vi "Teleop.vi"(10 "Match Info":T2={"Autonomous Elapsed Seconds"=0.0, "TeleOp Elapsed Seconds"=0.0, "Disabled Elapsed Seconds"=0.0, "Visited Autonomous"=FALSE, "Visited TeleOp"=FALSE, "Visited Disabled"=FALSE, "Autonomous Settings"={"Autonomous Style"=enum."Independent", "VI Refnum"=refnum}}, 11 "Call Context":T3) -> ()   [LabVIEW 2017]
doc: "This VI is called for each TeleOp packet received from the DS where the robot is not disabled. It is often used to read from the joysticks and update I/O or to update setpoints for timed control loops. It should complete and return within 20 milliseconds or it may miss DS packets."
uses:
  <vilib>/Rock Robotics/WPI/DriverStation/WPI_DriverStationDerivedRobotMode.ctl
  <vilib>/Rock Robotics/WPI/DriverStation/WPI_DriverStationMatch Info.ctl
  <vilib>/Rock Robotics/WPI/Solenoid/WPI_SolenoidValue.ctl
  <vilib>/Rock Robotics/WPI/Utilities/WPI_GetSetVariantRefNum.vi
  <vilib>/Rock Robotics/WPI/Solenoid/WPI_SolenoidSetEnum.vi
  <vilib>/Rock Robotics/WPI/RobotDrive/WPI_RobotDriveMecanumDrive_Cartesian.vi
  <vilib>/Rock Robotics/Network Tables/NT Write Numeric Array.vi
  <vilib>/Rock Robotics/Network Tables/NT Write Number.vi
  Robot Global Data.vi
panel:
  out "Stopped":bool
  out "Rate":dbl
  out "Direction":bool
  out "Distance":dbl
  out "Accelerations":T1
  out "Switch Pressed":bool
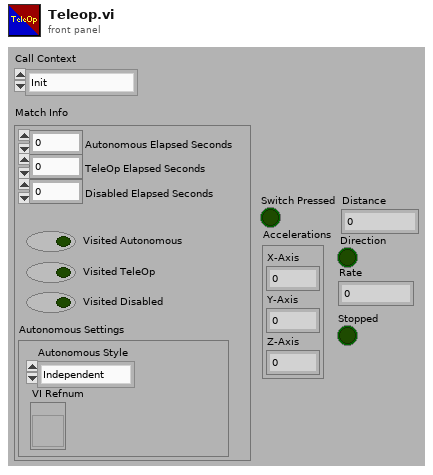
[diagram p1: front panel]
types:
  T1 = cluster{"X-Axis":dbl, "Y-Axis":dbl, "Z-Axis":dbl}
  T2 = typedef "WPI_DriverStationMatch Info.ctl" = cluster{"Autonomous Elapsed Seconds":dbl, "TeleOp Elapsed Seconds":dbl, "Disabled Elapsed Seconds":dbl, "Visited Autonomous":bool, "Visited TeleOp":bool, "Visited Disabled":bool, "Autonomous Settings":cluster{"Autonomous Style":enum16{"Iterative", "Independent"}, "VI Refnum":refnum<vi>}}
  T3 = typedef "WPI_DriverStationDerivedRobotMode.ctl" = enum16{"Init", "Execute", "Stop"}
  T4 = typedef "WPI_RobotDriveDevRef.ctl" = cluster{"DevStatus":errorcluster, "Motors[]":T5[], "Square Inputs":bool, "Max Output":dbl}
  T5 = typedef "WPI_MotorControlDeviceRef.ctl" = cluster{"DeviceStatus":errorcluster, "Type":T6, "PWM":cluster{"PWM Channel":T7, "DeadBand":T8}, "CAN":cluster{"Device Number":u8, "SetOutput VI Ref":variant, "GetOutput VI Ref":variant, "Enable VI Ref":variant, "Disable VI Ref":variant, "Data":variant}, "Invert":bool, "DIO PWM":cluster{"PWM \"Enable\" Channel":T7, "DIOChannel":T9, "PWM Rate":dbl}}
  T6 = typedef "WPI_MotorControlType.ctl" = enum16{"PWM", "CAN", "DIO PWM"}
  T7 = typedef "FPGA_DIOPWMChannel.ctl" = enum8{"PWM 0", "PWM 1", "PWM 2", "PWM 3", "PWM 4", "PWM 5", "PWM 6", "PWM 7", "PWM 8", "PWM 9", "PWM MXP 0", "PWM MXP 1", "PWM MXP 2", "PWM MXP 3", "PWM MXP 4", "PWM MXP 5", "PWM MXP 6", "PWM MXP 7", "PWM MXP 8", "PWM MXP 9", "Invalid"}
  T8 = typedef "WPI_PWMDeadband.ctl" = cluster{"Name":string, "maxPositivePwm":i32, "minPositivePwm":i32, "centerPwm":i32, "maxNegativePwm":i32, "minNegativePwm":i32, "angularRange":u16}
  T9 = typedef "FPGA_DIOChannel.ctl" = enum8{"DIO 0", "DIO 1", "DIO 2", "DIO 3", "DIO 4", "DIO 5", "DIO 6", "DIO 7", "DIO 8", "DIO 9", "DIO MXP 0", "DIO MXP 1", "DIO MXP 2", "DIO MXP 3", "DIO MXP 4", "DIO MXP 5", "DIO MXP 6", "DIO MXP 7", "DIO MXP 8", "DIO MXP 9", "DIO MXP 10", "DIO MXP 11", "DIO MXP 12", "DIO MXP 13", "DIO MXP 14", "DIO MXP 15", "SPI Port CS1", "SPI Port CS2", "SPI Port CS3", "SPI Port MISO", "SPI Port MOSI", "Invalid"}
  T10 = typedef "WPI_JoystickDevRef.ctl" = cluster{"Device":T11}
  T11 = typedef "WPI_JoystickDeviceEnum.ctl" = enum16{"USB 0", "USB 1", "USB 2", "USB 3", "USB 4", "USB 5"}
  T12 = typedef "WPI_SolenoidValue.ctl" = enum16{"Off", "On", "Forward", "Reverse"}
  T13 = typedef "WPI_SolenoidDevRef.ctl" = cluster{"DevStatus":errorcluster, "Pneumatics Control Module":u8, "Forward Solenoid Channel":T14, "Reverse Solenoid Channel":T14}
  T14 = typedef "WPI_SolenoidChannel.ctl" = enum8{"Solenoid 0", "Solenoid 1", "Solenoid 2", "Solenoid 3", "Solenoid 4", "Solenoid 5", "Solenoid 6", "Solenoid 7", "Invalid"}
  T15 = typedef "WPI_SwitchDevRef.ctl" = cluster{"DevStatus":errorcluster, "DIO Channel":T9, "CntIndex":T16, "Normally Closed":bool}
  T16 = typedef "FPGA_CounterCtrSystemIndex.ctl" = enum8{"Ctr 0", "Ctr 1", "Ctr 2", "Ctr 3", "Ctr 4", "Ctr 5", "Ctr 6", "Ctr 7", "Invalid"}
  T17 = typedef "WPI_AccelerometerDevRef.ctl" = cluster{"DevStatus":errorcluster, "Scaling":T18, "Analog Channels":T19, "I2C Bus":T21, "SPI Bus":T22, "Accel Range":T23, "ADXL Axes":T24, "Handle":i32, "Device Address":u8, "Accel Type":enum16{"Analog", "ADXL345 I2C", "ADXL345 SPI", "Internal", "ADXL362 SPI"}}
  T18 = typedef "WPI_AccelerometerScaling.ctl" = cluster{"Gain (VoltsPerG)":dbl, "Center Voltage":dbl}
  T19 = typedef "WPI_AccelerometerAnalogChannels.ctl" = cluster{"X-Axis":T20, "Y-Axis":T20, "Z-Axis":T20}
  T20 = typedef "FPGA_AIChannel.ctl" = enum8{"AI 0", "AI 1", "AI 2", "AI 3", "AI MXP 0", "AI MXP 1", "AI MXP 2", "AI MXP 3", "Invalid"}
  T21 = typedef "i2c_bus.ctl" = enum16{"I2C On-Board", "I2C MXP", "Invalid"}
  T22 = typedef "spi_bus.ctl" = enum16{"SPI On-Board, CS0", "SPI On-Board, CS1", "SPI On-Board, CS2", "SPI On-Board, CS3", "SPI MXP", "Invalid"}
  T23 = typedef "ADXL345 Range.ctl" = u8
  T24 = typedef "WPI_AccelerometerADXL345 Axes.ctl" = cluster{"X-Axis":bool, "Y-Axis":bool, "Z-Axis":bool}
  T25 = typedef "WPI_EncoderDevRef.ctl" = cluster{"DevStatus":errorcluster, "EncoderIndex":T26, "CounterIndex":T16, "DistancePerCount":dbl, "Decoding Type":T27}
  T26 = typedef "FPGA_EncoderIdx.ctl" = enum8{"Enc 0", "Enc 1", "Enc 2", "Enc 3", "Enc 4", "Enc 5", "Enc 6", "Enc 7", "Invalid"}
  T27 = typedef "WPI_EncoderType.ctl" = enum16{"1x", "2x", "4x"}
  T28 = typedef "WPI_GyroDevRef.ctl" = cluster{"DevStatus":errorcluster, "Analog Channel":T20, "Gain (VoltsPerDegree/Second)":dbl, "Gyro Type":enum16{"Analog", "XRS450"}, "Handle":i32, "SPI Bus":T22, "Device Found":bool, "Sample Rate":dbl, "Calibrate On Open":bool, "Offset":dbl}
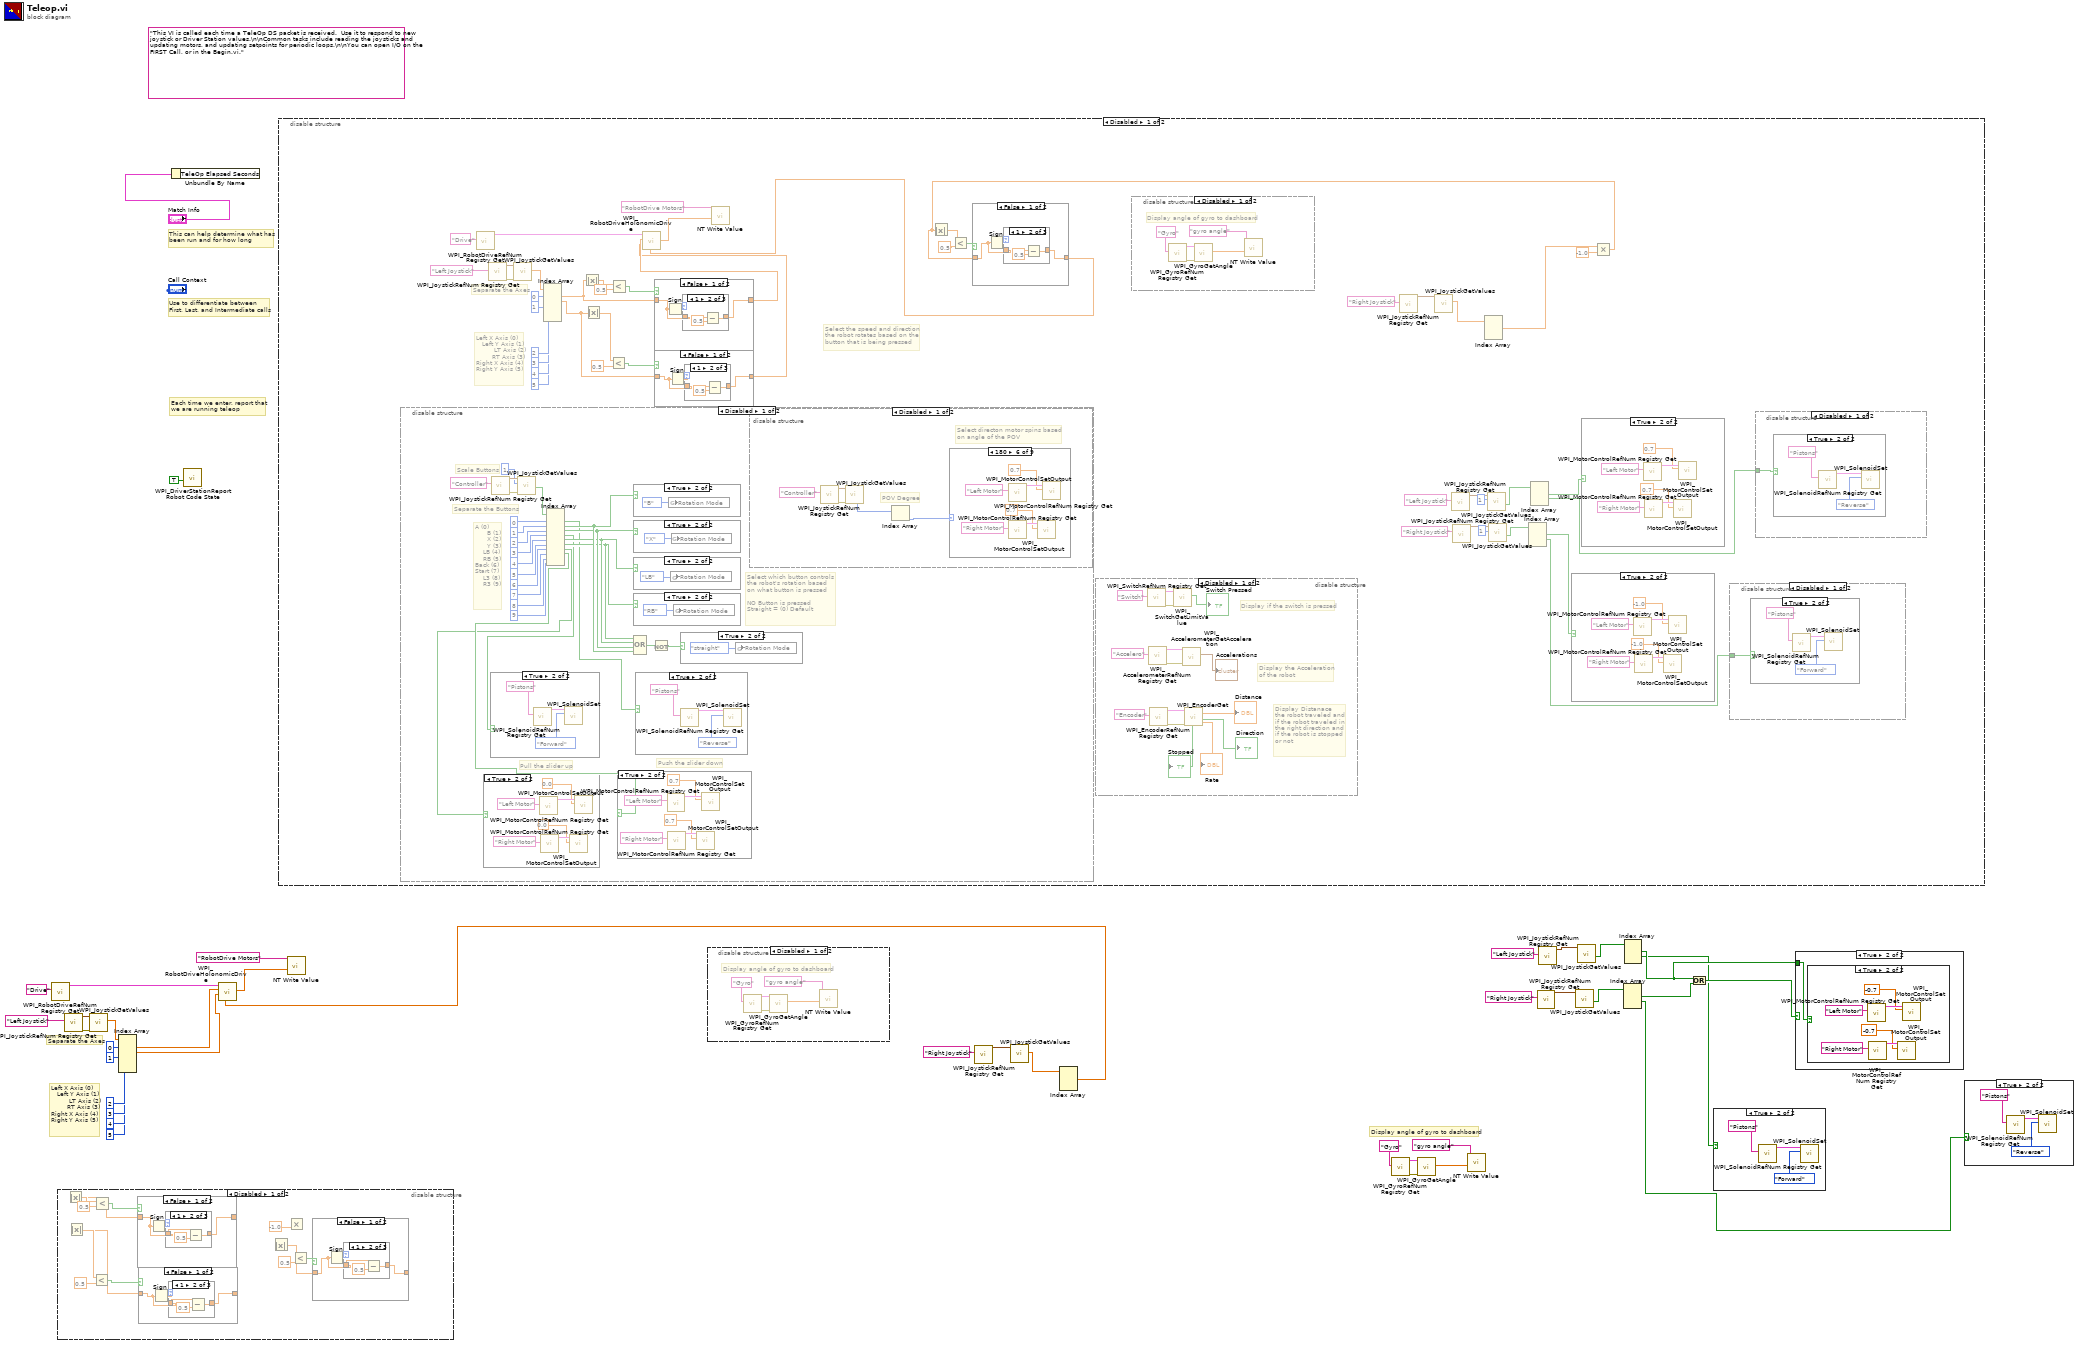
[diagram p0: block diagram]
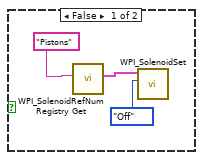
[diagram p2: hidden frame]
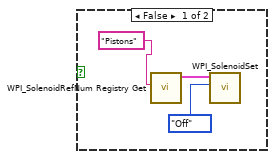
[diagram p3: hidden frame]
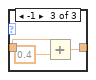
[diagram p5: hidden frame]
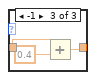
[diagram p8: hidden frame]
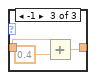
[diagram p11: hidden frame]
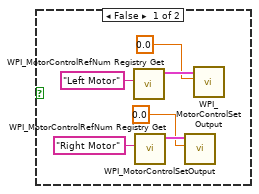
[diagram p15: hidden frame]
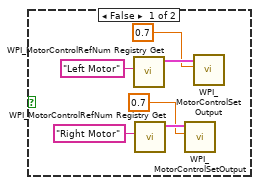
[diagram p16: hidden frame]
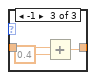
[diagram p18: hidden frame]
diagram:
  (unwired) "This VI is called each time a TeleOp DS packet is received.  Use it to respond to new joystick or Driver Station values.\n\nCommon tasks include reading the joysticks and updating motors, and updating setpoints for periodic loops.\n\nYou can open I/O on the FIRST Call, or in the Begin.vi."
  # "Display angle of gyro to dashboard"
  # "Left X Axis (0)\n   Left Y Axis (1)\n         LT Axis (2)\n        RT Axis (3)\nRight X Axis (4)\nRight Y Axis (5)"
  # "Separate the Axes"
  # "Each time we enter, report that\nwe are running teleop"
  # "Use to differentiate between\nFirst, Last, and Intermediate calls"
  # "This can help determine what has\nbeen run and for how long"
  n1 = call <vilib>:"WPI_RobotDriveRefNum Registry Get.vi"("refnum name"="Drive") -> ("RobotDriveDevRef"=w22:T4)  [unwired: 9 in, 1 out]
  n2 = disable-structure shown="Disabled" {
    frame Disabled {
      n3 = Absolute Value() -> (x=w45:dbl, abs(x)=w51:dbl)
      n4 = Absolute Value() -> (x=w44:dbl, abs(x)=w50:dbl)
      n5 = Less?(x=w50, y=0.5) -> (x < y?=w46:bool)
      n6 = Less?(x=w51, y=0.5) -> (x < y?=w47:bool)
      n7 = case shown="False" w47 {
        tunnel: [w74 w84] -> _
        tunnel: w45 -> [w75 w84]
        frame False {
          n8 = Sign(1:w75) -> (0:w76:dbl)
          n9 = case shown="1" w76 {
            tunnel: [w77 w80 w83] -> w74
            tunnel: w75 -> [w77 w78 w81]
            frame 0, Default {
            }
            frame 1 {
              n10 = Subtract(x=w78, y=0.5) -> (x-y=w80:dbl)
            }
            frame -1 {
              n11 = Add(x=w81, y=0.4) -> (x+y=w83:dbl)
            }
          }
        }
        frame True {
        }
      }
      n12 = case shown="False" w46 {
        tunnel: w44 -> [w64 w73]
        tunnel: [w63 w73] -> _
        frame False {
          n13 = Sign(1:w64) -> (0:w65:dbl)
          n14 = case shown="1" w65 {
            tunnel: [w66 w69 w72] -> w63
            tunnel: w64 -> [w66 w67 w70]
            frame 0, Default {
            }
            frame 1 {
              n15 = Subtract(x=w67, y=0.5) -> (x-y=w69:dbl)
            }
            frame -1 {
              n16 = Add(x=w70, y=0.4) -> (x+y=w72:dbl)
            }
          }
        }
        frame True {
        }
      }
      n17 = Absolute Value() -> (x=w43:dbl, abs(x)=w41:dbl)
      n18 = Multiply(y=-1.0) -> ()  [unwired: 1 in, 1 out]
      n19 = Less?(x=w41, y=0.5) -> (x < y?=w42:bool)
      n20 = case shown="False" w42 {
        tunnel: w43 -> [w53 w62]
        tunnel: [w52 w62] -> _
        frame False {
          n21 = Sign(1:w53) -> (0:w54:dbl)
          n22 = case shown="1" w54 {
            tunnel: [w55 w58 w61] -> w52
            tunnel: w53 -> [w55 w56 w59]
            frame 0, Default {
            }
            frame 1 {
              n23 = Subtract(x=w56, y=0.5) -> (x-y=w58:dbl)
            }
            frame -1 {
              n24 = Add(x=w59, y=0.4) -> (x+y=w61:dbl)
            }
          }
        }
        frame True {
        }
      }
    }
    frame Enabled {
    }
  }
  n25 = call <vilib>:"WPI_JoystickRefNum Registry Get.vi"("refnum name"="Left Joystick") -> ("error out"=w26:errorcluster, "JoystickDevRef"=w25:T10)  [unwired: 9 in]
  n26 = call <vilib>:"WPI_JoystickGetValues.vi"("error in (no error)"=w26, "JoystickDevRef"=w25) -> ("Axes"=w24:dbl[])  [unwired: 5 in, 4 out]
  n27 = Index Array(array=w24, index #1=0 ("index"), index #2=1 ("index"), index #3=2 ("index"), index #4=3 ("index"), index #5=4 ("index"), index #6=5 ("index")) -> (element #1=w5:dbl, element #2=w4:dbl)  [unwired: 4 out]
  n28 = Unbundle By Name("Match Info") -> ()  [unwired: 1 out]
  n29 = call <vilib>:"WPI_DriverStationReport Robot Code State.vi"("TeleOp"=TRUE ("Autonomous")) -> ()  [unwired: 10 in, 1 out]
  n30 = disable-structure shown="Disabled" {
    frame Disabled {
      # "Select the speed and direction\nthe robot rotates based on the \nbutton that is being pressed"
      # "Left X Axis (0)\n   Left Y Axis (1)\n         LT Axis (2)\n        RT Axis (3)\nRight X Axis (4)\nRight Y Axis (5)"
      # "Separate the Axes"
      n31 = disable-structure shown="Disabled" {
        frame Disabled {
          # "Select which button controls\nthe robot's rotation based\non what button is pressed\n\nNO Button is pressed\nStraight = (0) Default"
          # "Pull the slider up"
          # "Push the slider down"
          # "A (0)\n      B (1)\n      X (2)\n      Y (3)\n    LB (4)\n    RB (5)\nBack (6)\nStart (7)\n    L3 (8)\n    R3 (9)"
          # "Separate the Buttons"
          # "Scale Buttons"
          n32 = call <vilib>:"WPI_JoystickRefNum Registry Get.vi"("refnum name"="Controller") -> ("error out"=w226:errorcluster, "JoystickDevRef"=w225:T10)  [unwired: 9 in]
          n33 = call <vilib>:"WPI_JoystickGetValues.vi"("error in (no error)"=w226, "Scaler"=i8 1, "JoystickDevRef"=w225) -> ("Buttons"=w204:bool[])  [unwired: 4 in, 4 out]
          n34 = Index Array(array=w204, index #1=0 ("index"), index #2=1 ("index"), index #3=2 ("index"), index #4=3 ("index"), index #5=4 ("index"), index #6=5 ("index"), index #7=6 ("index"), index #8=7 ("index"), index #9=8 ("index"), index #10=9 ("index")) -> (element #1=w206:bool, element #2=w210:bool, element #3=w209:bool, element #4=w205:bool, element #5=w208:bool, element #6=w207:bool, element #7=w202:bool, element #8=w203:bool)  [unwired: 2 out]
          n35 = case shown="True" w202 {
            frame False {
            }
            frame True {
              n36 = call <vilib>:"WPI_MotorControlRefNum Registry Get.vi"("refnum name"="Left Motor") -> ("MotorControlDevRef"=w237:T5)  [unwired: 9 in, 1 out]
              n37 = call <vilib>:"WPI_MotorControlRefNum Registry Get.vi"("refnum name"="Right Motor") -> ("MotorControlDevRef"=w238:T5)  [unwired: 9 in, 1 out]
              n38 = call <vilib>:"WPI_MotorControlSetOutput.vi"("Output"=0.0, "MotorControlDevRef"=w238) -> ()  [unwired: 7 in, 3 out]
              n39 = call <vilib>:"WPI_MotorControlSetOutput.vi"("Output"=0.0, "MotorControlDevRef"=w237) -> ()  [unwired: 7 in, 3 out]
            }
          }
          n40 = case shown="True" w205 {
            frame False {
              n41 = call <vilib>:"WPI_SolenoidRefNum Registry Get.vi"("refnum name"="Pistons") -> ("SolenoidDevRef"=w241:T13)  [unwired: 9 in, 1 out]
              n42 = call-poly <vilib>:"WPI_SolenoidSet.vi"("Value"=WPI_SolenoidValue."Off", "SolenoidDevRef"=w241) -> ()  [unwired: 8 in, 2 out]
            }
            frame True {
              n43 = call <vilib>:"WPI_SolenoidRefNum Registry Get.vi"("refnum name"="Pistons") -> ("SolenoidDevRef"=w243:T13)  [unwired: 9 in, 1 out]
              n44 = call-poly <vilib>:"WPI_SolenoidSet.vi"("Value"=WPI_SolenoidValue."Forward", "SolenoidDevRef"=w243) -> ()  [unwired: 8 in, 2 out]
            }
          }
          n45 = case shown="True" w203 {
            frame False {
            }
            frame True {
              n46 = call <vilib>:"WPI_MotorControlRefNum Registry Get.vi"("refnum name"="Left Motor") -> ("MotorControlDevRef"=w231:T5)  [unwired: 9 in, 1 out]
              n47 = call <vilib>:"WPI_MotorControlRefNum Registry Get.vi"("refnum name"="Right Motor") -> ("MotorControlDevRef"=w229:T5)  [unwired: 9 in, 1 out]
              n48 = call <vilib>:"WPI_MotorControlSetOutput.vi"("Output"=0.7, "MotorControlDevRef"=w229) -> ()  [unwired: 7 in, 3 out]
              n49 = call <vilib>:"WPI_MotorControlSetOutput.vi"("Output"=0.7, "MotorControlDevRef"=w231) -> ()  [unwired: 7 in, 3 out]
            }
          }
          n50 = Compound Arithmetic op=OR(w207, w208, w209, w210) -> (w222:bool)
          n51 = case shown="True" w210 {
            frame False {
            }
            frame True {
              n52 = global write "Robot Global Data.vi" "Rotation Mode"(enum16{"straight", "X", "LB", "B", "RB"}."B" ("Rotation Mode")) -> ()
            }
          }
          n53 = case shown="True" w209 {
            frame False {
            }
            frame True {
              n54 = global write "Robot Global Data.vi" "Rotation Mode"(enum16{"straight", "X", "LB", "B", "RB"}."X" ("Rotation Mode")) -> ()
            }
          }
          n55 = case shown="True" w208 {
            frame False {
            }
            frame True {
              n56 = global write "Robot Global Data.vi" "Rotation Mode"(enum16{"straight", "X", "LB", "B", "RB"}."LB" ("Rotation Mode")) -> ()
            }
          }
          n57 = case shown="True" w207 {
            frame False {
            }
            frame True {
              n58 = global write "Robot Global Data.vi" "Rotation Mode"(enum16{"straight", "X", "LB", "B", "RB"}."RB" ("Rotation Mode")) -> ()
            }
          }
          n59 = case shown="True" w206 {
            frame False {
              n60 = call <vilib>:"WPI_SolenoidRefNum Registry Get.vi"("refnum name"="Pistons") -> ("SolenoidDevRef"=w247:T13)  [unwired: 9 in, 1 out]
              n61 = call-poly <vilib>:"WPI_SolenoidSet.vi"("Value"=WPI_SolenoidValue."Off", "SolenoidDevRef"=w247) -> ()  [unwired: 8 in, 2 out]
            }
            frame True {
              n62 = call <vilib>:"WPI_SolenoidRefNum Registry Get.vi"("refnum name"="Pistons") -> ("SolenoidDevRef"=w249:T13)  [unwired: 9 in, 1 out]
              n63 = call-poly <vilib>:"WPI_SolenoidSet.vi"("Value"=WPI_SolenoidValue."Reverse", "SolenoidDevRef"=w249) -> ()  [unwired: 8 in, 2 out]
            }
          }
          n64 = Not(x=w222) -> (.not. x?=w221:bool)
          n65 = case shown="True" w221 {
            frame False {
            }
            frame True {
              n66 = global write "Robot Global Data.vi" "Rotation Mode"(enum16{"straight", "X", "LB", "B", "RB"}."straight" ("Rotation Mode")) -> ()
            }
          }
          n67 = disable-structure shown="Disabled" {
            frame Disabled {
              # "Select directon motor spins based\non angle of the POV"
              # "POV Degree"
              n68 = call <vilib>:"WPI_JoystickRefNum Registry Get.vi"("refnum name"="Controller") -> ("error out"=w260:errorcluster, "JoystickDevRef"=w259:T10)  [unwired: 9 in]
              n69 = call <vilib>:"WPI_JoystickGetValues.vi"("error in (no error)"=w260, "JoystickDevRef"=w259) -> ("POVs"=w257:i16[])  [unwired: 5 in, 4 out]
              n70 = Index Array(array=w257) -> (element=w256:i16)  [unwired: 1 in]
              n71 = case shown="180" w256 {
                frame 0 {
                  n72 = call <vilib>:"WPI_MotorControlRefNum Registry Get.vi"("refnum name"="Left Motor") -> ("MotorControlDevRef"=w265:T5)  [unwired: 9 in, 1 out]
                  n73 = call <vilib>:"WPI_MotorControlRefNum Registry Get.vi"("refnum name"="Right Motor") -> ("MotorControlDevRef"=w263:T5)  [unwired: 9 in, 1 out]
                  n74 = call <vilib>:"WPI_MotorControlSetOutput.vi"("Output"=-0.7, "MotorControlDevRef"=w263) -> ()  [unwired: 7 in, 3 out]
                  n75 = call <vilib>:"WPI_MotorControlSetOutput.vi"("Output"=-0.7, "MotorControlDevRef"=w265) -> ()  [unwired: 7 in, 3 out]
                }
                frame -1, Default {
                  n76 = call <vilib>:"WPI_MotorControlRefNum Registry Get.vi"("refnum name"="Left Motor") -> ("MotorControlDevRef"=w271:T5)  [unwired: 9 in, 1 out]
                  n77 = call <vilib>:"WPI_MotorControlRefNum Registry Get.vi"("refnum name"="Right Motor") -> ("MotorControlDevRef"=w269:T5)  [unwired: 9 in, 1 out]
                  n78 = call <vilib>:"WPI_MotorControlSetOutput.vi"("Output"=0.0, "MotorControlDevRef"=w269) -> ()  [unwired: 7 in, 3 out]
                  n79 = call <vilib>:"WPI_MotorControlSetOutput.vi"("Output"=0.0, "MotorControlDevRef"=w271) -> ()  [unwired: 7 in, 3 out]
                }
                frame 45 {
                }
                frame 90 {
                  n80 = call <vilib>:"WPI_MotorControlRefNum Registry Get.vi"("refnum name"="Left Motor") -> ("MotorControlDevRef"=w277:T5)  [unwired: 9 in, 1 out]
                  n81 = call <vilib>:"WPI_MotorControlRefNum Registry Get.vi"("refnum name"="Right Motor") -> ("MotorControlDevRef"=w275:T5)  [unwired: 9 in, 1 out]
                  n82 = call <vilib>:"WPI_MotorControlSetOutput.vi"("Output"=1.0, "MotorControlDevRef"=w275) -> ()  [unwired: 7 in, 3 out]
                  n83 = call <vilib>:"WPI_MotorControlSetOutput.vi"("Output"=-1.0, "MotorControlDevRef"=w277) -> ()  [unwired: 7 in, 3 out]
                }
                frame 135 {
                }
                frame 180 {
                  n84 = call <vilib>:"WPI_MotorControlRefNum Registry Get.vi"("refnum name"="Left Motor") -> ("MotorControlDevRef"=w283:T5)  [unwired: 9 in, 1 out]
                  n85 = call <vilib>:"WPI_MotorControlRefNum Registry Get.vi"("refnum name"="Right Motor") -> ("MotorControlDevRef"=w281:T5)  [unwired: 9 in, 1 out]
                  n86 = call <vilib>:"WPI_MotorControlSetOutput.vi"("Output"=0.7, "MotorControlDevRef"=w281) -> ()  [unwired: 7 in, 3 out]
                  n87 = call <vilib>:"WPI_MotorControlSetOutput.vi"("Output"=0.7, "MotorControlDevRef"=w283) -> ()  [unwired: 7 in, 3 out]
                }
                frame 225 {
                }
                frame 270 {
                  n88 = call <vilib>:"WPI_MotorControlRefNum Registry Get.vi"("refnum name"="Left Motor") -> ("MotorControlDevRef"=w289:T5)  [unwired: 9 in, 1 out]
                  n89 = call <vilib>:"WPI_MotorControlRefNum Registry Get.vi"("refnum name"="Right Motor") -> ("MotorControlDevRef"=w287:T5)  [unwired: 9 in, 1 out]
                  n90 = call <vilib>:"WPI_MotorControlSetOutput.vi"("Output"=-1.0, "MotorControlDevRef"=w287) -> ()  [unwired: 7 in, 3 out]
                  n91 = call <vilib>:"WPI_MotorControlSetOutput.vi"("Output"=1.0, "MotorControlDevRef"=w289) -> ()  [unwired: 7 in, 3 out]
                }
                frame 315 {
                }
              }
            }
            frame Enabled {
            }
          }
        }
        frame Enabled {
        }
      }
      n92 = call <vilib>:"WPI_RobotDriveRefNum Registry Get.vi"("refnum name"="Drive") -> ("RobotDriveDevRef"=w125:T4)  [unwired: 9 in, 1 out]
      n93 = call <vilib>:"WPI_JoystickRefNum Registry Get.vi"("refnum name"="Left Joystick") -> ("error out"=w129:errorcluster, "JoystickDevRef"=w128:T10)  [unwired: 9 in]
      n94 = call <vilib>:"WPI_JoystickGetValues.vi"("error in (no error)"=w129, "JoystickDevRef"=w128) -> ("Axes"=w127:dbl[])  [unwired: 5 in, 4 out]
      n95 = Index Array(array=w127, index #1=0 ("index"), index #2=1 ("index"), index #3=2 ("index"), index #4=3 ("index"), index #5=4 ("index"), index #6=5 ("index")) -> (element #1=w93:dbl, element #2=w92:dbl)  [unwired: 4 out]
      n96 = Absolute Value(x=w93) -> (abs(x)=w99:dbl)
      n97 = Absolute Value(x=w92) -> (abs(x)=w98:dbl)
      n98 = Less?(x=w98, y=0.5) -> (x < y?=w94:bool)
      n99 = Less?(x=w99, y=0.5) -> (x < y?=w95:bool)
      n100 = case shown="False" w95 {
        tunnel: [w153 w163] -> w91
        tunnel: w93 -> [w154 w163]
        frame False {
          n101 = Sign(1:w154) -> (0:w155:dbl)
          n102 = case shown="1" w155 {
            tunnel: [w156 w159 w162] -> w153
            tunnel: w154 -> [w156 w157 w160]
            frame 0, Default {
            }
            frame 1 {
              n103 = Subtract(x=w157, y=0.5) -> (x-y=w159:dbl)
            }
            frame -1 {
              n104 = Add(x=w160, y=0.4) -> (x+y=w162:dbl)
            }
          }
        }
        frame True {
        }
      }
      n105 = case shown="False" w94 {
        tunnel: w92 -> [w143 w152]
        tunnel: [w142 w152] -> w90
        frame False {
          n106 = Sign(1:w143) -> (0:w144:dbl)
          n107 = case shown="1" w144 {
            tunnel: [w145 w148 w151] -> w142
            tunnel: w143 -> [w145 w146 w149]
            frame 0, Default {
            }
            frame 1 {
              n108 = Subtract(x=w146, y=0.5) -> (x-y=w148:dbl)
            }
            frame -1 {
              n109 = Add(x=w149, y=0.4) -> (x+y=w151:dbl)
            }
          }
        }
        frame True {
        }
      }
      n110 = disable-structure shown="Disabled" {
        frame Disabled {
          # "Display Distanace\nthe robot traveled and\nif the robot traveled in \nthe right direction and\nif the robot is stopped \nor not"
          # "Display the Acceleration\nof the robot"
          # "Display if the switch is pressed"
          n111 = call <vilib>:"WPI_SwitchRefNum Registry Get.vi"("refnum name"="Switch") -> ("error out"=w309:errorcluster, "SwitchDevRef"=w308:T15)  [unwired: 9 in]
          n112 = call <vilib>:"WPI_AccelerometerRefNum Registry Get.vi"("refnum name"="Accelero") -> ("error out"=w306:errorcluster, "AccelerometerDevRef"=w305:T17)  [unwired: 9 in]
          n113 = call <vilib>:"WPI_EncoderRefNum Registry Get.vi"("refnum name"="Encoder") -> ("error out"=w301:errorcluster, "EncoderDevRef"=w300:T25)  [unwired: 9 in]
          n114 = call <vilib>:"WPI_SwitchGetLimitValue.vi"("error in (no error)"=w309, "SwitchDevRef"=w308) -> ("Switch Pressed"=→"Switch Pressed":bool)  [unwired: 7 in, 2 out]
          n115 = call <vilib>:"WPI_AccelerometerGetAcceleration.vi"("error in"=w306, "AccelerometerDevRef"=w305) -> ("Accelerations"=→"Accelerations":T1)  [unwired: 7 in, 2 out]
          n116 = call <vilib>:"WPI_EncoderGet.vi"("error in (no error)"=w301, "EncoderDevRef"=w300) -> ("Direction"=→"Direction":bool, "Distance"=→"Distance":dbl, "Rate"=→"Rate":dbl, "Stopped"=→"Stopped":bool)  [unwired: 4 in, 2 out]
        }
        frame Enabled {
        }
      }
      n117 = disable-structure shown="Disabled" {
        frame Disabled {
          # "Display angle of gyro to dashboard"
          n118 = call <vilib>:"WPI_GyroRefNum Registry Get.vi"("refnum name"="Gyro") -> ("error out"=w294:errorcluster, "GyroDevRef"=w293:T28)  [unwired: 9 in]
          n119 = call <vilib>:"WPI_GyroGetAngle.vi"("error in"=w294, "GyroDevRef"=w293) -> ("Angle"=w291:dbl)  [unwired: 5 in, 4 out]
          n120 = call-poly <vilib>:"NT Write Value.vi"("Numeric"=w291, "Name"="gyro angle") -> ()  [unwired: 9 in, 1 out]
        }
        frame Enabled {
        }
      }
      n121 = call <vilib>:"WPI_JoystickRefNum Registry Get.vi"("refnum name"="Right Joystick") -> ("JoystickDevRef"=w115:T10)  [unwired: 9 in, 1 out]
      n122 = call <vilib>:"WPI_JoystickGetValues.vi"("JoystickDevRef"=w115) -> ("Axes"=w114:dbl[])  [unwired: 6 in, 4 out]
      n123 = call <vilib>:"WPI_JoystickRefNum Registry Get.vi"("refnum name"="Left Joystick") -> ("JoystickDevRef"=w110:T10)  [unwired: 9 in, 1 out]
      n124 = call <vilib>:"WPI_JoystickRefNum Registry Get.vi"("refnum name"="Right Joystick") -> ("JoystickDevRef"=w112:T10)  [unwired: 9 in, 1 out]
      n125 = Index Array(array=w114) -> (element #1=w100:dbl)  [unwired: 3 in, 2 out]
      n126 = call <vilib>:"WPI_JoystickGetValues.vi"("Scaler"=i8 1, "JoystickDevRef"=w110) -> ("Buttons"=w107:bool[])  [unwired: 5 in, 4 out]
      n127 = call <vilib>:"WPI_JoystickGetValues.vi"("Scaler"=i8 1, "JoystickDevRef"=w112) -> ("Buttons"=w106:bool[])  [unwired: 5 in, 4 out]
      n128 = Index Array(array=w106) -> (element #1=w105:bool, element #2=w102:bool)  [unwired: 3 in, 1 out]
      n129 = Index Array(array=w107) -> (element #1=w104:bool, element #2=w103:bool)  [unwired: 3 in, 1 out]
      n130 = case shown="True" w105 {
        frame False {
          n131 = call <vilib>:"WPI_MotorControlRefNum Registry Get.vi"("refnum name"="Left Motor") -> ("MotorControlDevRef"=w194:T5)  [unwired: 9 in, 1 out]
          n132 = call <vilib>:"WPI_MotorControlRefNum Registry Get.vi"("refnum name"="Right Motor") -> ("MotorControlDevRef"=w195:T5)  [unwired: 9 in, 1 out]
          n133 = call <vilib>:"WPI_MotorControlSetOutput.vi"("Output"=0.0, "MotorControlDevRef"=w195) -> ()  [unwired: 7 in, 3 out]
          n134 = call <vilib>:"WPI_MotorControlSetOutput.vi"("Output"=0.0, "MotorControlDevRef"=w194) -> ()  [unwired: 7 in, 3 out]
        }
        frame True {
          n135 = call <vilib>:"WPI_MotorControlRefNum Registry Get.vi"("refnum name"="Left Motor") -> ("MotorControlDevRef"=w200:T5)  [unwired: 9 in, 1 out]
          n136 = call <vilib>:"WPI_MotorControlRefNum Registry Get.vi"("refnum name"="Right Motor") -> ("MotorControlDevRef"=w198:T5)  [unwired: 9 in, 1 out]
          n137 = call <vilib>:"WPI_MotorControlSetOutput.vi"("Output"=-1.0, "MotorControlDevRef"=w198) -> ()  [unwired: 7 in, 3 out]
          n138 = call <vilib>:"WPI_MotorControlSetOutput.vi"("Output"=-1.0, "MotorControlDevRef"=w200) -> ()  [unwired: 7 in, 3 out]
        }
      }
      n139 = case shown="True" w104 {
        frame False {
          n140 = call <vilib>:"WPI_MotorControlRefNum Registry Get.vi"("refnum name"="Left Motor") -> ("MotorControlDevRef"=w182:T5)  [unwired: 9 in, 1 out]
          n141 = call <vilib>:"WPI_MotorControlRefNum Registry Get.vi"("refnum name"="Right Motor") -> ("MotorControlDevRef"=w183:T5)  [unwired: 9 in, 1 out]
          n142 = call <vilib>:"WPI_MotorControlSetOutput.vi"("Output"=0.0, "MotorControlDevRef"=w183) -> ()  [unwired: 7 in, 3 out]
          n143 = call <vilib>:"WPI_MotorControlSetOutput.vi"("Output"=0.0, "MotorControlDevRef"=w182) -> ()  [unwired: 7 in, 3 out]
        }
        frame True {
          n144 = call <vilib>:"WPI_MotorControlRefNum Registry Get.vi"("refnum name"="Left Motor") -> ("MotorControlDevRef"=w188:T5)  [unwired: 9 in, 1 out]
          n145 = call <vilib>:"WPI_MotorControlRefNum Registry Get.vi"("refnum name"="Right Motor") -> ("MotorControlDevRef"=w186:T5)  [unwired: 9 in, 1 out]
          n146 = call <vilib>:"WPI_MotorControlSetOutput.vi"("Output"=0.7, "MotorControlDevRef"=w186) -> ()  [unwired: 7 in, 3 out]
          n147 = call <vilib>:"WPI_MotorControlSetOutput.vi"("Output"=0.7, "MotorControlDevRef"=w188) -> ()  [unwired: 7 in, 3 out]
        }
      }
      n148 = Multiply(x=w100, y=-1.0) -> (x*y=w86:dbl)
      n149 = Absolute Value(x=w86) -> (abs(x)=w89:dbl)
      n150 = Less?(x=w89, y=0.5) -> (x < y?=w87:bool)
      n151 = case shown="False" w87 {
        tunnel: w86 -> [w132 w141]
        tunnel: [w131 w141] -> w85
        frame False {
          n152 = Sign(1:w132) -> (0:w133:dbl)
          n153 = case shown="1" w133 {
            tunnel: [w134 w137 w140] -> w131
            tunnel: w132 -> [w134 w135 w138]
            frame 0, Default {
            }
            frame 1 {
              n154 = Subtract(x=w135, y=0.5) -> (x-y=w137:dbl)
            }
            frame -1 {
              n155 = Add(x=w138, y=0.4) -> (x+y=w140:dbl)
            }
          }
        }
        frame True {
        }
      }
      n156 = call-poly <vilib>:"WPI_RobotDriveHolonomicDrive.vi"("Rotation"=w85, "Y"=w90, "X"=w91, "RobotDriveDevRef"=w125) -> ("Motor Values"=w124:dbl[])  [unwired: 5 in, 2 out]
      n157 = call-poly <vilib>:"NT Write Value.vi"("Numeric Array"=w124, "Name"="RobotDrive Motors") -> ()  [unwired: 9 in, 1 out]
      n158 = disable-structure shown="Disabled" {
        disable-tunnel: w102 -> [w164 _]
        frame Disabled {
          n159 = case shown="True" w164 {
            frame False {
              n160 = call <vilib>:"WPI_SolenoidRefNum Registry Get.vi"("refnum name"="Pistons") -> ("SolenoidDevRef"=w167:T13)  [unwired: 9 in, 1 out]
              n161 = call-poly <vilib>:"WPI_SolenoidSet.vi"("Value"=WPI_SolenoidValue."Off", "SolenoidDevRef"=w167) -> ()  [unwired: 8 in, 2 out]
            }
            frame True {
              n162 = call <vilib>:"WPI_SolenoidRefNum Registry Get.vi"("refnum name"="Pistons") -> ("SolenoidDevRef"=w169:T13)  [unwired: 9 in, 1 out]
              n163 = call-poly <vilib>:"WPI_SolenoidSet.vi"("Value"=WPI_SolenoidValue."Forward", "SolenoidDevRef"=w169) -> ()  [unwired: 8 in, 2 out]
            }
          }
        }
        frame Enabled {
        }
      }
      n164 = disable-structure shown="Disabled" {
        disable-tunnel: w103 -> [w171 _]
        frame Disabled {
          n165 = case shown="True" w171 {
            frame False {
              n166 = call <vilib>:"WPI_SolenoidRefNum Registry Get.vi"("refnum name"="Pistons") -> ("SolenoidDevRef"=w174:T13)  [unwired: 9 in, 1 out]
              n167 = call-poly <vilib>:"WPI_SolenoidSet.vi"("Value"=WPI_SolenoidValue."Off", "SolenoidDevRef"=w174) -> ()  [unwired: 8 in, 2 out]
            }
            frame True {
              n168 = call <vilib>:"WPI_SolenoidRefNum Registry Get.vi"("refnum name"="Pistons") -> ("SolenoidDevRef"=w176:T13)  [unwired: 9 in, 1 out]
              n169 = call-poly <vilib>:"WPI_SolenoidSet.vi"("Value"=WPI_SolenoidValue."Reverse", "SolenoidDevRef"=w176) -> ()  [unwired: 8 in, 2 out]
            }
          }
        }
        frame Enabled {
        }
      }
    }
    frame Enabled {
    }
  }
  n170 = disable-structure shown="Disabled" {
    frame Disabled {
      # "Display angle of gyro to dashboard"
      n171 = call <vilib>:"WPI_GyroRefNum Registry Get.vi"("refnum name"="Gyro") -> ("error out"=w314:errorcluster, "GyroDevRef"=w313:T28)  [unwired: 9 in]
      n172 = call <vilib>:"WPI_GyroGetAngle.vi"("error in"=w314, "GyroDevRef"=w313) -> ("Angle"=w311:dbl)  [unwired: 5 in, 4 out]
      n173 = call-poly <vilib>:"NT Write Value.vi"("Numeric"=w311, "Name"="gyro angle") -> ()  [unwired: 9 in, 1 out]
    }
    frame Enabled {
    }
  }
  n174 = call <vilib>:"WPI_JoystickRefNum Registry Get.vi"("refnum name"="Right Joystick") -> ("JoystickDevRef"=w12:T10)  [unwired: 9 in, 1 out]
  n175 = call <vilib>:"WPI_JoystickGetValues.vi"("JoystickDevRef"=w12) -> ("Axes"=w11:dbl[])  [unwired: 6 in, 4 out]
  n176 = Index Array(array=w11) -> (element #1=w3:dbl)  [unwired: 3 in, 2 out]
  n177 = call-poly <vilib>:"WPI_RobotDriveHolonomicDrive.vi"("Rotation"=w3, "Y"=w4, "X"=w5, "RobotDriveDevRef"=w22) -> ("Motor Values"=w21:dbl[])  [unwired: 5 in, 2 out]
  n178 = call-poly <vilib>:"NT Write Value.vi"("Numeric Array"=w21, "Name"="RobotDrive Motors") -> ()  [unwired: 9 in, 1 out]
  n179 = call <vilib>:"WPI_GyroRefNum Registry Get.vi"("refnum name"="Gyro") -> ("error out"=w9:errorcluster, "GyroDevRef"=w8:T28)  [unwired: 9 in]
  n180 = call <vilib>:"WPI_GyroGetAngle.vi"("error in"=w9, "GyroDevRef"=w8) -> ("Angle"=w6:dbl)  [unwired: 5 in, 4 out]
  n181 = call-poly <vilib>:"NT Write Value.vi"("Numeric"=w6, "Name"="gyro angle") -> ()  [unwired: 9 in, 1 out]
  n182 = call <vilib>:"WPI_JoystickRefNum Registry Get.vi"("refnum name"="Right Joystick") -> ("JoystickDevRef"=w36:T10)  [unwired: 9 in, 1 out]
  n183 = call <vilib>:"WPI_JoystickRefNum Registry Get.vi"("refnum name"="Left Joystick") -> ("JoystickDevRef"=w35:T10)  [unwired: 9 in, 1 out]
  n184 = call <vilib>:"WPI_JoystickGetValues.vi"("JoystickDevRef"=w36) -> ("Buttons"=w33:bool[])  [unwired: 6 in, 4 out]
  n185 = call <vilib>:"WPI_JoystickGetValues.vi"("JoystickDevRef"=w35) -> ("Buttons"=w34:bool[])  [unwired: 6 in, 4 out]
  n186 = Index Array(array=w33) -> (element #1=w30:bool, element #2=w1:bool)  [unwired: 3 in, 1 out]
  n187 = Index Array(array=w34) -> (element #1=w28:bool, element #2=w2:bool)  [unwired: 3 in, 1 out]
  n188 = Or(x=w28, y=w30) -> (x .or. y?=w29:bool)
  n189 = case shown="True" w2 {
    frame False {
      n190 = call <vilib>:"WPI_SolenoidRefNum Registry Get.vi"("refnum name"="Pistons") -> ("SolenoidDevRef"=w318:T13)  [unwired: 9 in, 1 out]
      n191 = call-poly <vilib>:"WPI_SolenoidSet.vi"("Value"=WPI_SolenoidValue."Off", "SolenoidDevRef"=w318) -> ()  [unwired: 8 in, 2 out]
    }
    frame True {
      n192 = call <vilib>:"WPI_SolenoidRefNum Registry Get.vi"("refnum name"="Pistons") -> ("SolenoidDevRef"=w320:T13)  [unwired: 9 in, 1 out]
      n193 = call-poly <vilib>:"WPI_SolenoidSet.vi"("Value"=WPI_SolenoidValue."Forward", "SolenoidDevRef"=w320) -> ()  [unwired: 8 in, 2 out]
    }
  }
  n194 = case shown="True" w29 {
    tunnel: w28 -> [_ w328]
    frame False {
      n195 = call <vilib>:"WPI_MotorControlRefNum Registry Get.vi"("refnum name"="Left Motor") -> ("MotorControlDevRef"=w326:T5)  [unwired: 9 in, 1 out]
      n196 = call <vilib>:"WPI_MotorControlRefNum Registry Get.vi"("refnum name"="Right Motor") -> ("MotorControlDevRef"=w324:T5)  [unwired: 9 in, 1 out]
      n197 = call <vilib>:"WPI_MotorControlSetOutput.vi"("Output"=0.0, "MotorControlDevRef"=w324) -> ()  [unwired: 7 in, 3 out]
      n198 = call <vilib>:"WPI_MotorControlSetOutput.vi"("Output"=0.0, "MotorControlDevRef"=w326) -> ()  [unwired: 7 in, 3 out]
    }
    frame True {
      n199 = case shown="True" w328 {
        frame False {
          n200 = call <vilib>:"WPI_MotorControlRefNum Registry Get.vi"("refnum name"="Left Motor") -> ("MotorControlDevRef"=w333:T5)  [unwired: 9 in, 1 out]
          n201 = call <vilib>:"WPI_MotorControlRefNum Registry Get.vi"("refnum name"="Right Motor") -> ("MotorControlDevRef"=w331:T5)  [unwired: 9 in, 1 out]
          n202 = call <vilib>:"WPI_MotorControlSetOutput.vi"("Output"=0.7, "MotorControlDevRef"=w331) -> ()  [unwired: 7 in, 3 out]
          n203 = call <vilib>:"WPI_MotorControlSetOutput.vi"("Output"=0.7, "MotorControlDevRef"=w333) -> ()  [unwired: 7 in, 3 out]
        }
        frame True {
          n204 = call <vilib>:"WPI_MotorControlRefNum Registry Get.vi"("refnum name"="Left Motor") -> ("MotorControlDevRef"=w339:T5)  [unwired: 9 in, 1 out]
          n205 = call <vilib>:"WPI_MotorControlRefNum Registry Get.vi"("refnum name"="Right Motor") -> ("MotorControlDevRef"=w337:T5)  [unwired: 9 in, 1 out]
          n206 = call <vilib>:"WPI_MotorControlSetOutput.vi"("Output"=-0.7, "MotorControlDevRef"=w337) -> ()  [unwired: 7 in, 3 out]
          n207 = call <vilib>:"WPI_MotorControlSetOutput.vi"("Output"=-0.7, "MotorControlDevRef"=w339) -> ()  [unwired: 7 in, 3 out]
        }
      }
    }
  }
  n208 = case shown="True" w1 {
    frame False {
      n209 = call <vilib>:"WPI_SolenoidRefNum Registry Get.vi"("refnum name"="Pistons") -> ("SolenoidDevRef"=w343:T13)  [unwired: 9 in, 1 out]
      n210 = call-poly <vilib>:"WPI_SolenoidSet.vi"("Value"=WPI_SolenoidValue."Off", "SolenoidDevRef"=w343) -> ()  [unwired: 8 in, 2 out]
    }
    frame True {
      n211 = call <vilib>:"WPI_SolenoidRefNum Registry Get.vi"("refnum name"="Pistons") -> ("SolenoidDevRef"=w345:T13)  [unwired: 9 in, 1 out]
      n212 = call-poly <vilib>:"WPI_SolenoidSet.vi"("Value"=WPI_SolenoidValue."Reverse", "SolenoidDevRef"=w345) -> ()  [unwired: 8 in, 2 out]
    }
  }
